vi "Save Image.vi"(8 "error in (no error)":errorcluster, 10 "Path":path, 11 "Optris PI in":refnum<class "Optris PI.lvclass">) -> (0 "error out":errorcluster, 3 "Optris PI out":refnum<class "Optris PI.lvclass">)   [LabVIEW 2018, in "Optris PI.lvlib" / "Optris PI.lvclass"]
uses:
  Optris PI.lvclass
  Optris PI.lvclass/Optris PI.ctl
  <instrlib>/Optris PI/libirimager_direct_binding.lvlib
  PPLs/Thermal Camera/Parent/Thermal Camera.lvlibp/Thermal Camera.lvclass
  C:/AME Test Engineering/LabVIEW/PPLs/Thermal Camera/Parent/Thermal Camera.lvlibp/Thermal Camera.lvclass
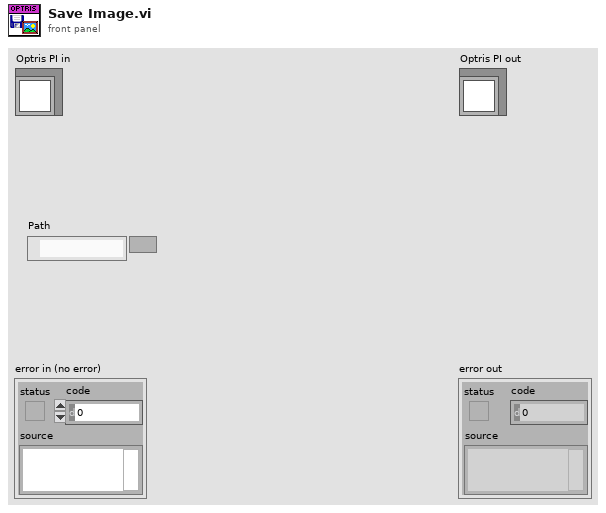
[diagram p1: front panel]
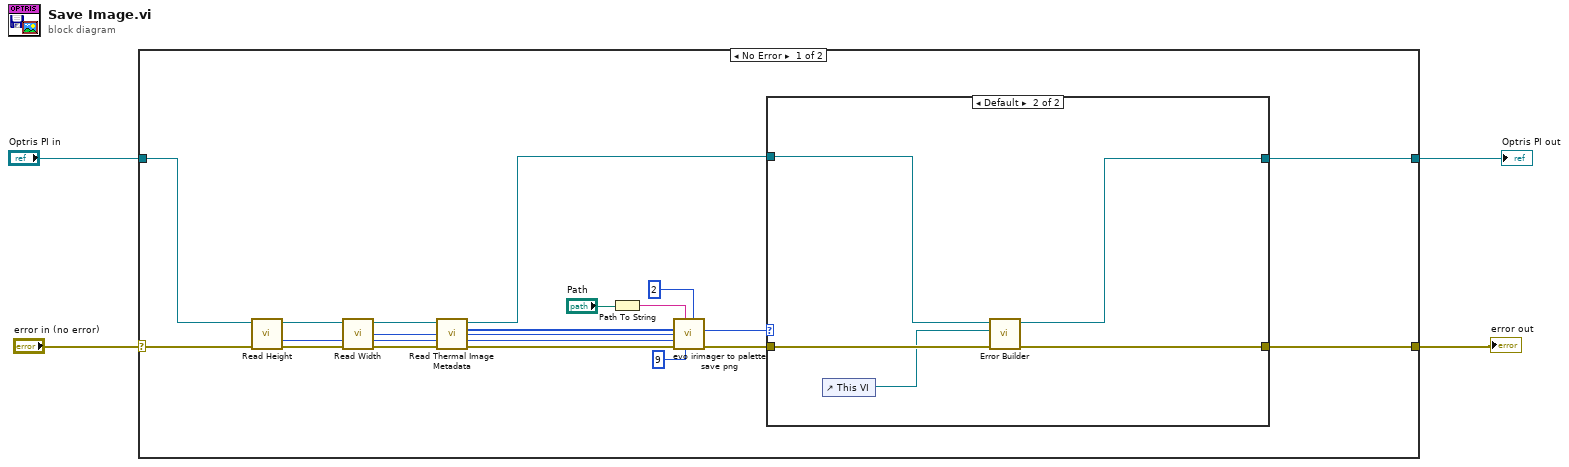
[diagram p0: block diagram]
diagram:
  n1 = case shown="No Error" "error in (no error)" {
    selector: "error in (no error)" -> [w16 w31]
    tunnel: [w6 w32] -> w3
    tunnel: "Optris PI in" -> [w17 w32]
    tunnel: [w5 w31] -> w1
    frame No Error {
      n2 = call "Read Height.vi"("error in (no error)"=w16, "Thermal Camera in"=w17) -> ("error out"=w14:errorcluster, "Height"=w10:u32, "Thermal Camera out"=w15:refnum<class "Optris PI.lvclass">)  [unwired: 7 in]
      n3 = call "Read Width.vi"("error in (no error)"=w14, "Thermal Camera in"=w15) -> ("error out"=w12:errorcluster, "Width"=w11:u32, "Thermal Camera out"=w13:refnum<class "Optris PI.lvclass">)  [unwired: 7 in]
      n4 = call "Read Thermal Image Metadata.vi"("error in (no error)"=w12, "Optris PI in"=w13) -> ("error out"=w22:errorcluster, "Thermal Image Metadata"=w23:u16[], "Optris PI out"=w8:refnum<class "Optris PI.lvclass">)  [unwired: 7 in]
      n5 = Path To String(path="Path") -> (string=w20:string)
      n6 = call <instrlib>:"evo irimager to palette save png.vi"("palette_scale"=2, "palette"=9, "path"=w20, "error in (no error)"=w22, "h"=w10, "w"=w11, "thermal_data"=w23) -> ("error out"=w7:errorcluster, "function return"=w9:i32)  [unwired: 2 in, 1 out]
      n7 = case shown="Default" w9 {
        tunnel: w8 -> [w25 w30]
        tunnel: w7 -> [w24 w29]
        tunnel: [w25 w28] -> w6
        tunnel: [w24 w27] -> w5
        frame 0 {
        }
        frame Default {
          n8 = control-ref of="This VI"() -> (w26:refnum<vi>)
          n9 = call "Error Builder.vi"("error in (no error)"=w29, "This VI"=w26, "Optris PI in"=w30) -> ("Error out"=w27:errorcluster, "Optris PI out"=w28:refnum<class "Optris PI.lvclass">)  [unwired: 7 in]
        }
      }
    }
    frame Error {
    }
  }
  "error out" <- w1
  "Optris PI out" <- w3
